vi "Const File Create.vi"() -> ()   [LabVIEW 2024]
uses:
  controls/Serial - Settings.ctl
  controls/Cal Sensor Enum.ctl
  <vilib>/Utility/config.llb/Write Key (String).vi
  <vilib>/Utility/config.llb/NI_LVConfig.lvlib
panel:
  in  "Value 7":T1
  in  "Calibration Sensor":T2
  out "success":bool
  out "error out 2":errorcluster
  in  "Value 6":T3
  in  "Value 5":T4
  in  "Value 4":T5
  in  "Value 3":T6
  in  "Value 2":T8 {"Port Settings"."flow control" items=["None"=0, "XON/XOFF"=1, "RTS/CTS"=2, "DTR/DSR"=4]; "Port Settings"."stop bits" items=["1.0"=10, "1.5"=15, "2.0"=20]; "Port Settings"."data bits" min=5 max=8 step=1; "Port Settings"."baud rate" items=["75"=75, "110"=110, "134"=134, "150"=150, "300"=300, "600"=600, "1200"=1200, "1800"=1800, "2400"=2400, "4800"=4800, "7200"=7200, "9600"=9600, "14400"=14400, "19200"=19200, "28800"=28800, "38400"=38400, "56000"=56000, "57600"=57600, "115200"=115200, "128000"=128000, "230400"=230400]}
  in  "Value":T9
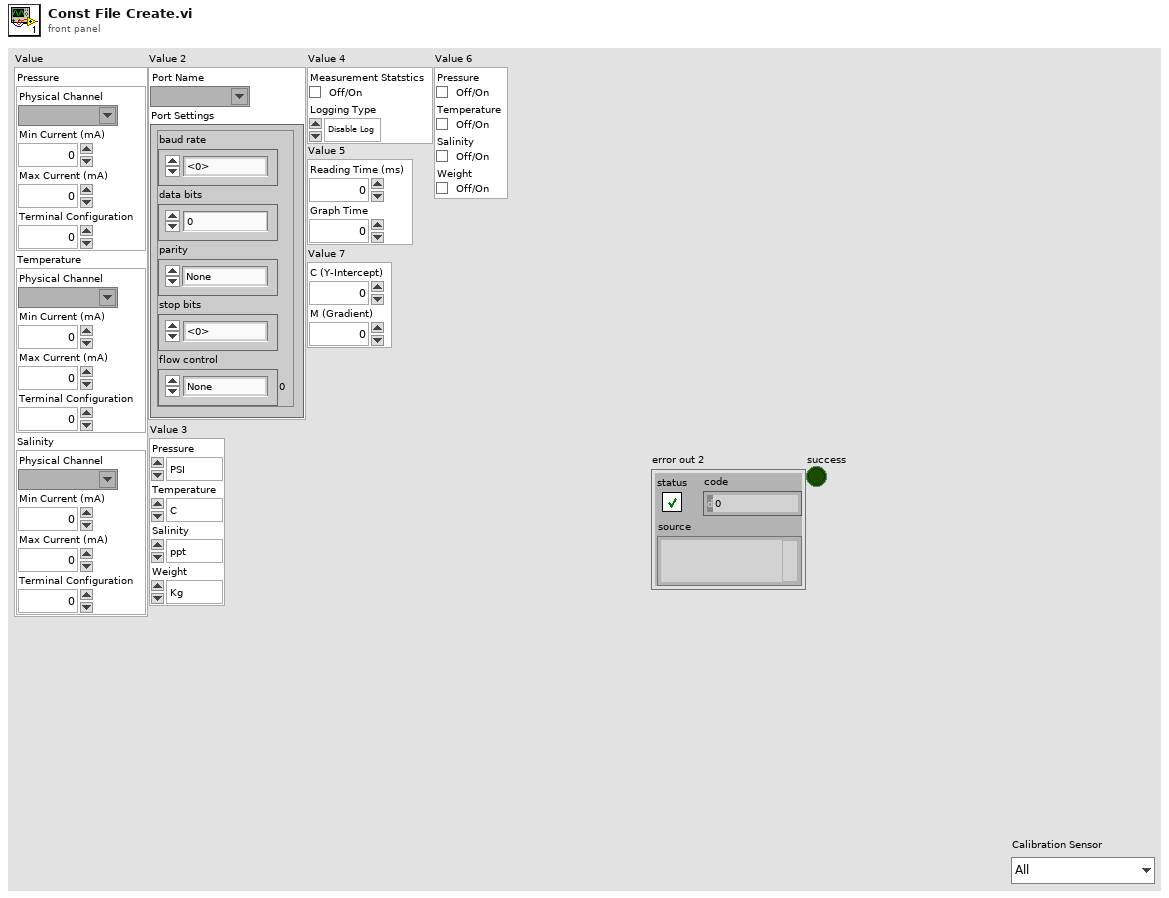
[diagram p1: front panel]
types:
  T1 = cluster{"C (Y-Intercept)":dbl, "M (Gradient)":dbl}
  T2 = typedef "Cal Sensor Enum.ctl" = enum16{"All", "Pressure", "Temperature", "Salinity", "Weight"}
  T3 = cluster{"Pressure":bool, "Temperature":bool, "Salinity":bool, "Weight":bool}
  T4 = cluster{"Reading Time (ms)":u64, "Graph Time ":u16}
  T5 = cluster{"Measurement Statstics":bool, "Logging Type":enum16{"Disable Log", "TDMS", "CSV"}}
  T6 = cluster{"Pressure":enum16{"PSI", "Bar", "atm", "Pa"}, "Temperature":enum16{"C", "K", "F"}, "Salinity":enum16{"ppt", "PSU"}, "Weight":enum16{"Kg", "g", "oz", "ib"}}
  T7 = typedef "Serial - Settings.ctl" = cluster{"baud rate":u32, "data bits":u16, "parity":enum16{"None", "Odd", "Even", "Mark", "Space"}, "stop bits":u16, "flow control":u16}
  T8 = cluster{"Port Name":refnum<visa-resource-name>, "Port Settings":T7}
  T9 = cluster{"Pressure":cluster{"Physical Channel":tag, "Min Current (mA)":dbl, "Max Current (mA)":dbl, "Terminal Configuration":i32}, "Temperature":cluster{"Physical Channel":tag, "Min Current (mA)":dbl, "Max Current (mA)":dbl, "Terminal Configuration":i32}, "Salinity":cluster{"Physical Channel":tag, "Min Current (mA)":dbl, "Max Current (mA)":dbl, "Terminal Configuration":i32}}
  T10 = typedef "NI_LVConfig.lvlib/Config Data RefNum.ctl" = refnum<k1>
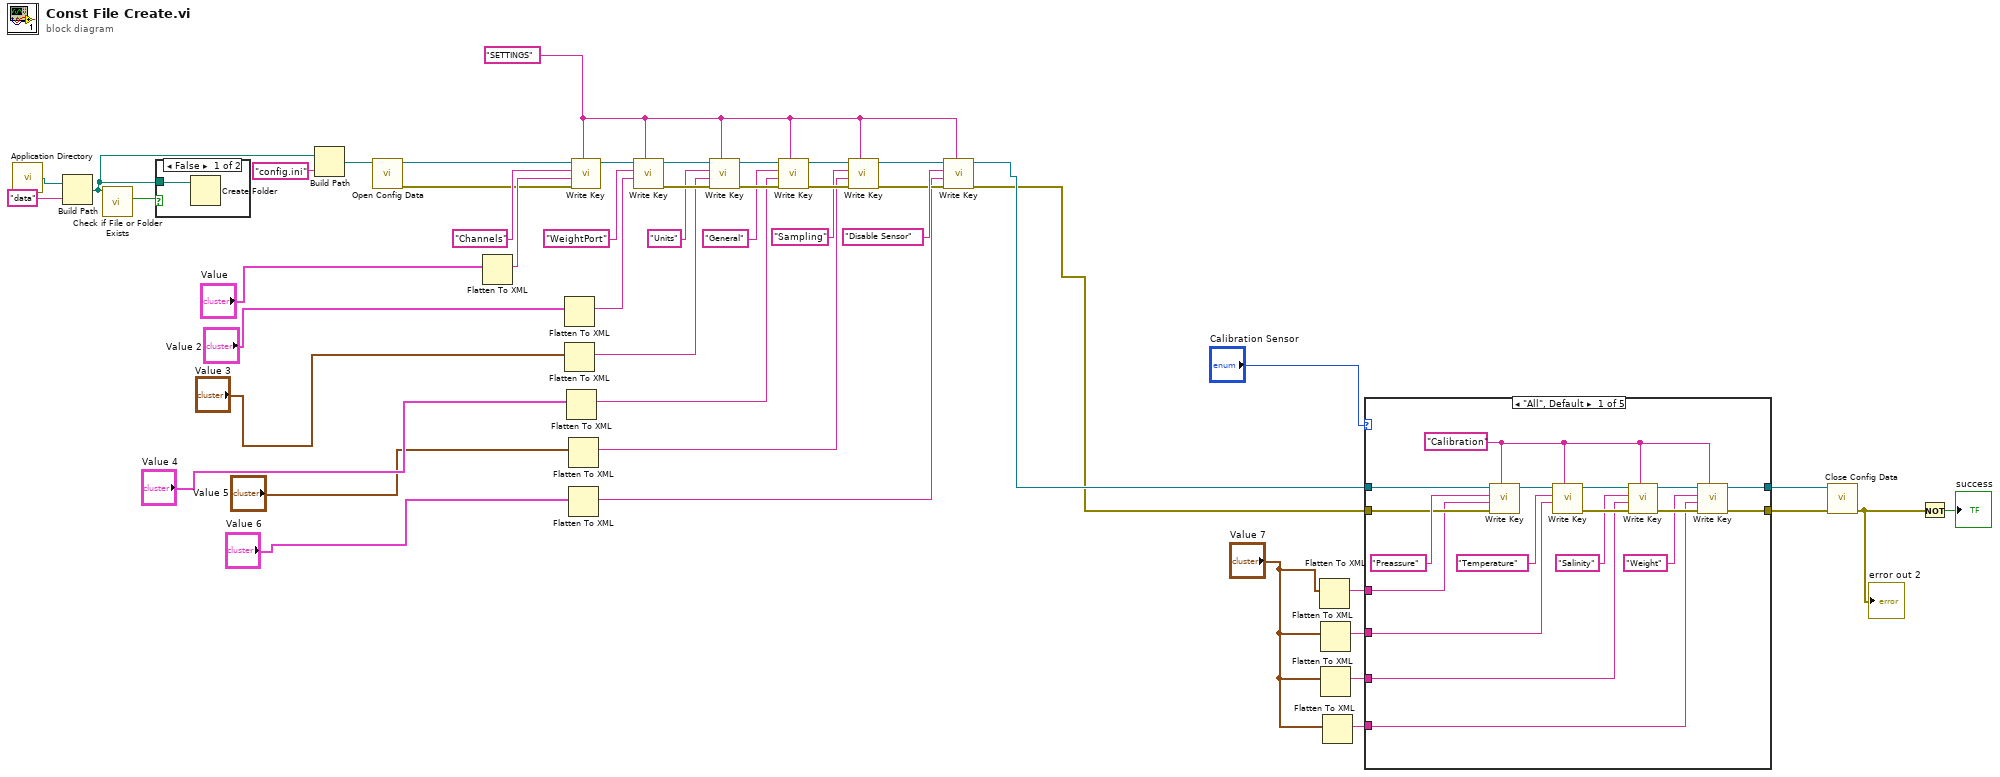
[diagram p0: block diagram]
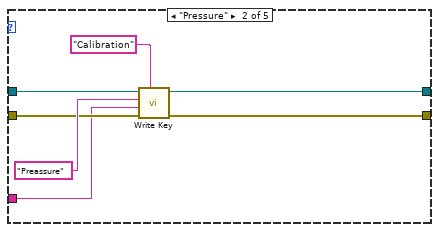
[diagram p2: hidden frame]
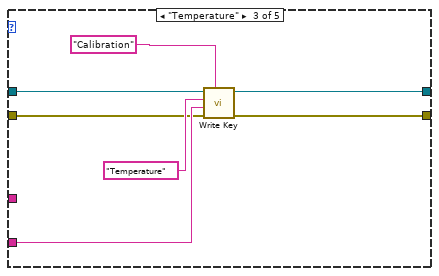
[diagram p3: hidden frame]
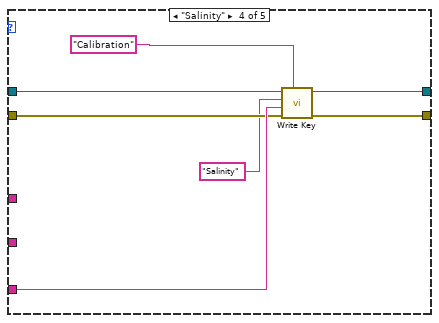
[diagram p4: hidden frame]
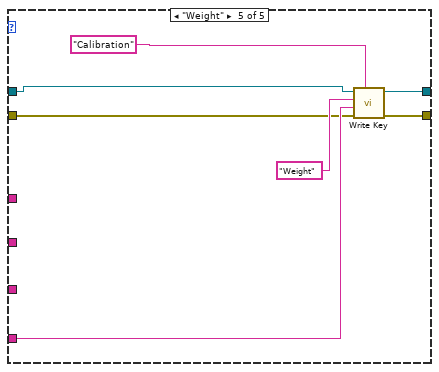
[diagram p5: hidden frame]
diagram:
  w27 = "SETTINGS" ("section")
  n1 = call <vilib>:"Application Directory.vi"() -> ("Application Directory"=w15:path)
  n2 = Build Path(base path=w15, name or relative path="data") -> (appended path=w13:path)
  n3 = call <vilib>:"Check if File or Folder Exists.vi"("path"=w13) -> ("file or folder exists?"=w14:bool)  [unwired: 8 in, 2 out]
  n4 = case shown="False" w14 {
    tunnel: w13 -> [w49 _]
    frame False {
      n5 = Create Folder(path (use dialog)=w49) -> ()  [unwired: 2 in, 3 out]
    }
    frame True {
    }
  }
  n6 = Build Path(base path=w13, name or relative path="config.ini") -> (appended path=w25:path)
  n7 = call <vilib>:"Open Config Data.vi"("configuration file path"=w25) -> ("error out"=w23:errorcluster, "refnum"=w24:T10)  [unwired: 8 in, 1 out]
  n8 = Flatten To XML(6:"Value") -> (2:w46:string)
  n9 = Flatten To XML(6:"Value 2") -> (2:w43:string)
  n10 = Flatten To XML(6:"Value 3") -> (2:w33:string)
  n11 = Flatten To XML(6:"Value 4") -> (2:w32:string)
  n12 = Flatten To XML(6:"Value 5") -> (2:w31:string)
  n13 = Flatten To XML(6:"Value 6") -> (2:w26:string)
  n14 = call-poly <vilib>:"Write Key.vi"("section"=w27, "error in (no error)"=w23, "value"=w46, "key"="Channels", "refnum"=w24) -> ("refnum out"=w44:T10)  [unwired: 4 in, 2 out]
  n15 = call-poly <vilib>:"Write Key.vi"("section"=w27, "value"=w43, "key"="WeightPort", "refnum"=w44) -> ("error out"=w41:errorcluster, "refnum out"=w42:T10)  [unwired: 5 in, 1 out]
  n16 = call-poly <vilib>:"Write Key.vi"("section"=w27, "error in (no error)"=w41, "value"=w33, "key"="Units", "refnum"=w42) -> ("error out"=w39:errorcluster, "refnum out"=w40:T10)  [unwired: 4 in, 1 out]
  n17 = call-poly <vilib>:"Write Key.vi"("section"=w27, "error in (no error)"=w39, "value"=w32, "key"="General", "refnum"=w40) -> ("error out"=w37:errorcluster, "refnum out"=w38:T10)  [unwired: 4 in, 1 out]
  n18 = call-poly <vilib>:"Write Key.vi"("section"=w27, "error in (no error)"=w37, "value"=w31, "key"="Sampling", "refnum"=w38) -> ("error out"=w29:errorcluster, "refnum out"=w28:T10)  [unwired: 4 in, 1 out]
  n19 = call-poly <vilib>:"Write Key.vi"("section"=w27, "error in (no error)"=w29, "value"=w26, "key"="Disable Sensor", "refnum"=w28) -> ("error out"=w1:errorcluster, "refnum out"=w3:T10)  [unwired: 4 in, 1 out]
  n20 = Flatten To XML(6:"Value 7") -> (2:w10:string)
  n21 = Flatten To XML(6:"Value 7") -> (2:w9:string)
  n22 = Flatten To XML(6:"Value 7") -> (2:w8:string)
  n23 = Flatten To XML(6:"Value 7") -> (2:w7:string)
  n24 = case shown="\"All\", Default" "Calibration Sensor" {
    tunnel: w3 -> [w67 w74 w78 w84 w90]
    tunnel: w1 -> [w65 w72 w77 w83 w89]
    tunnel: w10 -> [w64 w71 _ _ _]
    tunnel: w9 -> [w61 _ w80 _ _]
    tunnel: w8 -> [w53 _ _ w87 _]
    tunnel: w7 -> [w52 _ _ _ w93]
    tunnel: [w51 w69 w75 w86 w92] -> w6
    tunnel: [w50 w68 w76 w85 w91] -> w5
    frame "All", Default {
      w56 = "Calibration" ("section")
      n25 = call-poly <vilib>:"Write Key.vi"("section"=w56, "error in (no error)"=w65, "value"=w64, "key"="Preassure", "refnum"=w67) -> ("refnum out"=w62:T10)  [unwired: 4 in, 2 out]
      n26 = call-poly <vilib>:"Write Key.vi"("section"=w56, "value"=w61, "key"="Temperature", "refnum"=w62) -> ("error out"=w59:errorcluster, "refnum out"=w60:T10)  [unwired: 5 in, 1 out]
      n27 = call-poly <vilib>:"Write Key.vi"("section"=w56, "error in (no error)"=w59, "value"=w53, "key"="Salinity", "refnum"=w60) -> ("error out"=w57:errorcluster, "refnum out"=w58:T10)  [unwired: 4 in, 1 out]
      n28 = call-poly <vilib>:"Write Key.vi"("section"=w56, "error in (no error)"=w57, "value"=w52, "key"="Weight", "refnum"=w58) -> ("error out"=w50:errorcluster, "refnum out"=w51:T10)  [unwired: 4 in, 1 out]
    }
    frame "Pressure" {
      n29 = call-poly <vilib>:"Write Key.vi"("section"="Calibration", "error in (no error)"=w72, "value"=w71, "key"="Preassure", "refnum"=w74) -> ("error out"=w68:errorcluster, "refnum out"=w69:T10)  [unwired: 4 in, 1 out]
    }
    frame "Temperature" {
      n30 = call-poly <vilib>:"Write Key.vi"("section"="Calibration", "error in (no error)"=w77, "value"=w80, "key"="Temperature", "refnum"=w78) -> ("error out"=w76:errorcluster, "refnum out"=w75:T10)  [unwired: 4 in, 1 out]
    }
    frame "Salinity" {
      n31 = call-poly <vilib>:"Write Key.vi"("section"="Calibration", "error in (no error)"=w83, "value"=w87, "key"="Salinity", "refnum"=w84) -> ("error out"=w85:errorcluster, "refnum out"=w86:T10)  [unwired: 4 in, 1 out]
    }
    frame "Weight" {
      n32 = call-poly <vilib>:"Write Key.vi"("section"="Calibration", "error in (no error)"=w89, "value"=w93, "key"="Weight", "refnum"=w90) -> ("error out"=w91:errorcluster, "refnum out"=w92:T10)  [unwired: 4 in, 1 out]
    }
  }
  n33 = call <vilib>:"Close Config Data.vi"("error in (no error)"=w5, "refnum"=w6) -> ("error out"=w12:errorcluster)  [unwired: 8 in, 1 out]
  "error out 2" <- w12
  n34 = Not(x=w12) -> (.not. x?=→"success":bool)
